vi "ImportMouse.vi"(8 "error in (no error)":errorcluster, 10 "Tuple":T1={"mouse_id"=1217.0, "mouse_gender"="male", "mouse_strain"="C57BL6/J", "mouse_dob"="", "mouse_dod"="", "mouse_notes"="", "headpost_date"=""}, 11 "Database in":refnum<class "Database.lvclass">) -> (0 "error out":errorcluster, 3 "Database out":refnum<class "Database.lvclass">)   [LabVIEW 2014, in "Database.lvclass"]
uses:
  Database.lvclass
  Database.lvclass/Database.ctl
  <vilib>/addons/database/NI_Database_API.lvlib
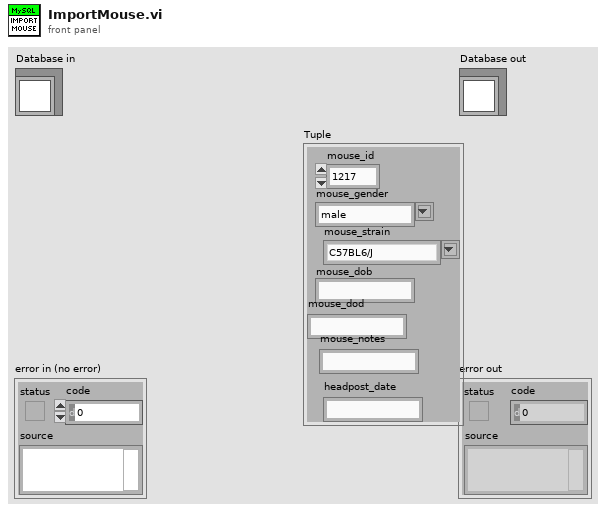
[diagram p1: front panel]
types:
  T1 = cluster{"mouse_id":dbl, "mouse_gender":string, "mouse_strain":string, "mouse_dob":string, "mouse_dod":string, "mouse_notes":string, "headpost_date":string}
  T2 = typedef "NI_Database_API.lvlib/Conn ObjectReference.ctl" = refnum<k1>
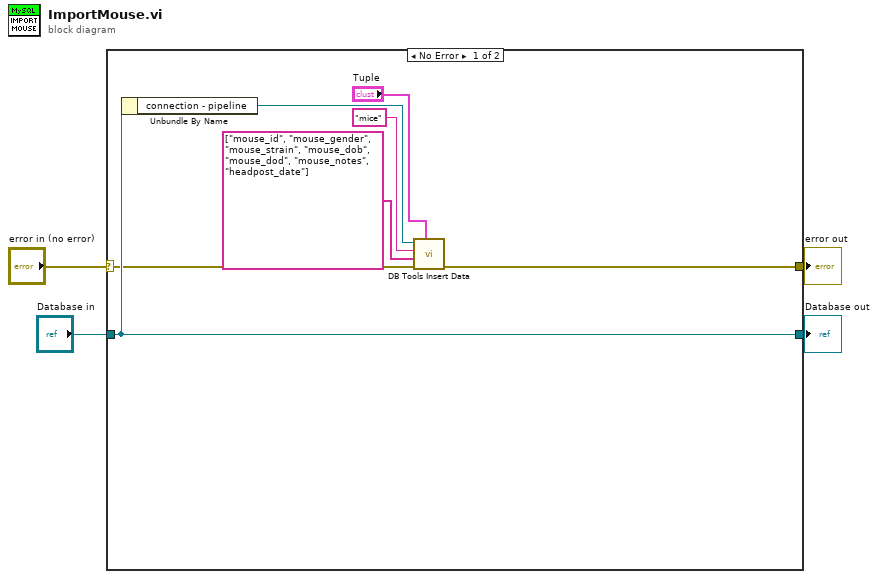
[diagram p0: block diagram]
diagram:
  n1 = case shown="No Error" "error in (no error)" {
    selector: "error in (no error)" -> [w7 w13]
    tunnel: [w6 w13] -> w3
    tunnel: [w8 w12] -> w1
    tunnel: "Database in" -> [w8 w12]
    frame No Error {
      n2 = Unbundle By Name(w8) -> ("connection - pipeline"=w10:T2)
      n3 = call <vilib>:"DB Tools Insert Data.vi"("data"="Tuple", "error in (no error)"=w7, "columns"=string[] ["mouse_id", "mouse_gender", "mouse_strain", "mouse_dob", "mouse_dod", "mouse_notes", "headpost_date"], "table"="mice", "connection reference"=w10) -> ("error out"=w6:errorcluster)  [unwired: 5 in, 1 out]
    }
    frame Error {
    }
  }
  "error out" <- w3
  "Database out" <- w1
